vi "Check Address Range.vi"(7 "Storage Size":i32, 8 "Length(Byte)":i32 format="%x", 9 "Offset":i32 format="%x", 10 "Page(hex)":i32 format="%x", 11 "Sector":i32) -> (2 "Address In Range":bool)   [LabVIEW 2012, in "NFC Driver.lvlib"]
uses:
  NFC Driver.lvlib
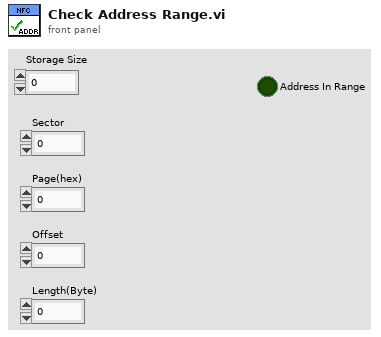
[diagram p1: front panel]
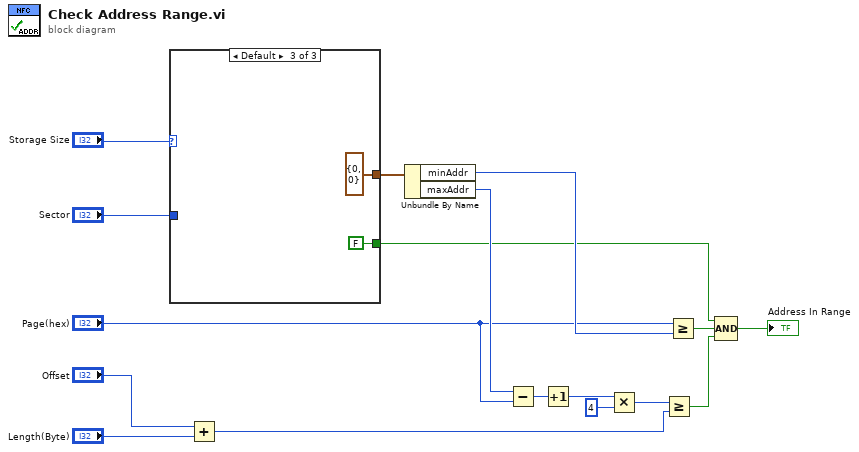
[diagram p0: block diagram]
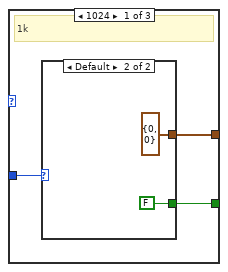
[diagram p2: hidden frame]
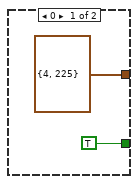
[diagram p3: hidden frame]
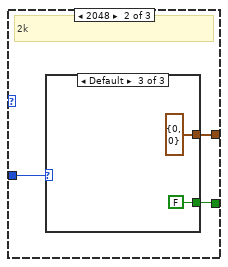
[diagram p4: hidden frame]
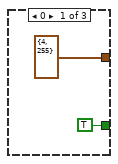
[diagram p5: hidden frame]
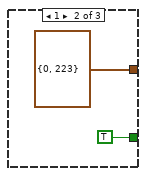
[diagram p6: hidden frame]
diagram:
  n1 = case shown="Default" "Storage Size" {
    tunnel: [w20 w27 cluster{"minAddr":i32, "maxAddr":i32} {"minAddr"=0, "maxAddr"=0}] -> w15
    tunnel: "Sector" -> [w19 w26 _]
    tunnel: [w18 w25 FALSE] -> w3
    frame 1024 {
      # "1k"
      n2 = case shown="Default" w19 {
        tunnel: [cluster{"minAddr":i32, "maxAddr":i32} {"minAddr"=4, "maxAddr"=225} cluster{"minAddr":i32, "maxAddr":i32} {"minAddr"=0, "maxAddr"=0}] -> w20
        tunnel: [TRUE FALSE] -> w18
        frame 0 {
        }
        frame Default {
        }
      }
    }
    frame 2048 {
      # "2k"
      n3 = case shown="Default" w26 {
        tunnel: [cluster{"minAddr":i32, "maxAddr":i32} {"minAddr"=4, "maxAddr"=255} cluster{"minAddr":i32, "maxAddr":i32} {"minAddr"=0, "maxAddr"=223} cluster{"minAddr":i32, "maxAddr":i32} {"minAddr"=0, "maxAddr"=0}] -> w27
        tunnel: [TRUE TRUE FALSE] -> w25
        frame 0 {
        }
        frame 1 {
        }
        frame Default {
        }
      }
    }
    frame Default {
    }
  }
  n4 = Add(x="Offset", y="Length(Byte)") -> (x+y=w8:i32)
  n5 = Unbundle By Name(w15) -> ("minAddr"=w14:i32, "maxAddr"=w13:i32)
  n6 = Subtract(x=w13, y="Page(hex)") -> (x-y=w11:i32)
  n7 = Increment(x=w11) -> (x+1=w1:i32)
  n8 = Multiply(x=w1, y=4) -> (x*y=w9:i32)
  n9 = Greater Or Equal?(x=w9, y=w8) -> (x >= y?=w5:bool)
  n10 = Greater Or Equal?(x="Page(hex)", y=w14) -> (x >= y?=w4:bool)
  n11 = Compound Arithmetic op=AND(w3, w4, w5) -> (→"Address In Range":bool)
